vi "Report PDFCreator.vi"(0 "report in":refnum<class "NI_report.lvclass">, 2 "Conversion to PDF":enum16{"standard report", "file"}(ring), 7 "AutosaveDirectory":string="C:\\Users\\A Blaise\\Desktop\\Alouette\\Documents BD\\Rapports\\", 9 "AutosaveFilename":string="Allo", 11 "error in (no error)":errorcluster, 13 "Printer name":string="PDFCreator") -> (4 "report out":refnum<class "NI_report.lvclass">, 8 "More than 60 seconds":bool, 10 "File path":path, 15 "error out":errorcluster)   [LabVIEW 2010]
doc: "Jean-Marc Simard \nJanuary 6, 2010"
uses:
  <vilib>/Utility/NIReport.llb/NI_report.lvclass
panel:
  in  "File to convert":path
  in  "PDFCreator._clsPDFCreator":refnum<k7>
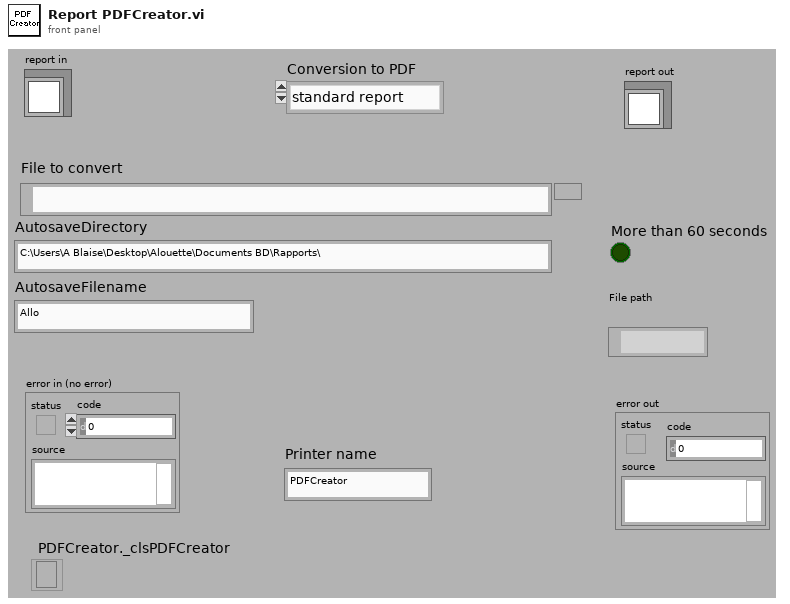
[diagram p1: front panel]
types:
  T1 = cluster{"UseAutosave":i32, "UseAutosaveDirectory":i32, "Autosave directory":string, "AutosaveFilename":string, "AutosaveFormat":i32}
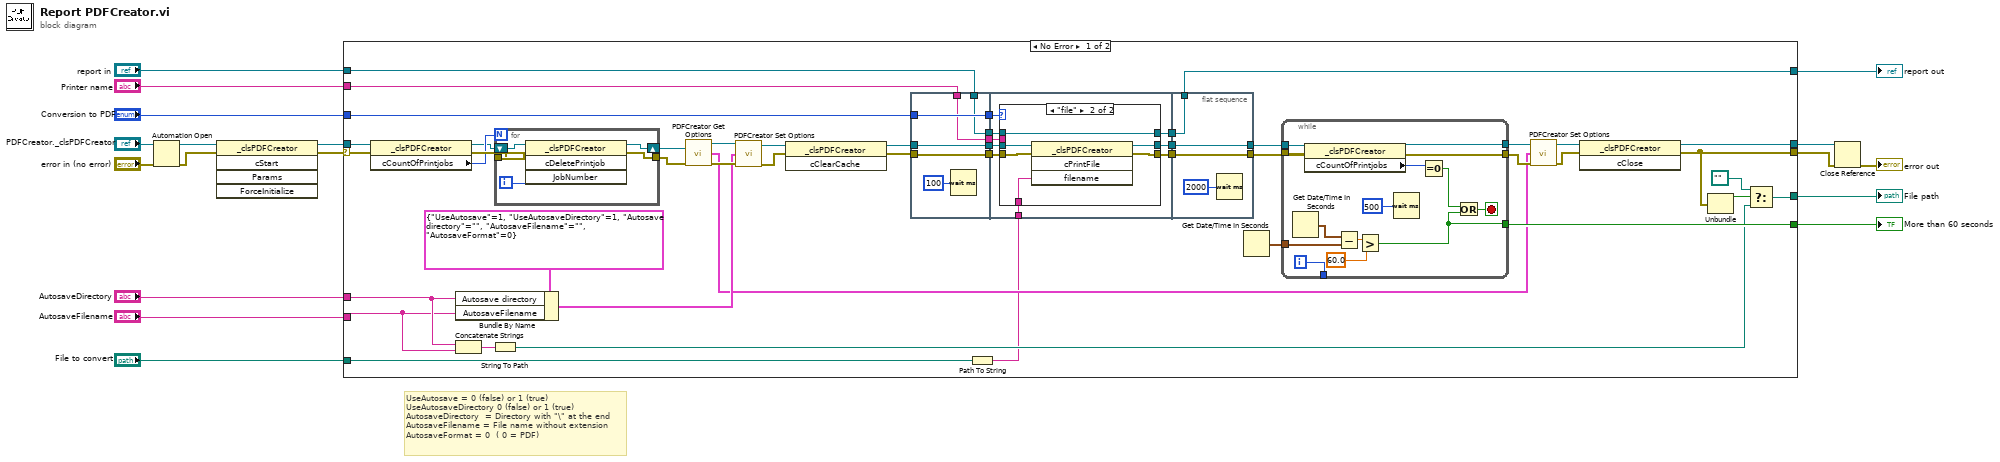
[diagram p0: block diagram]
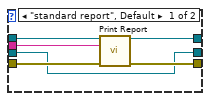
[diagram p2: hidden frame]
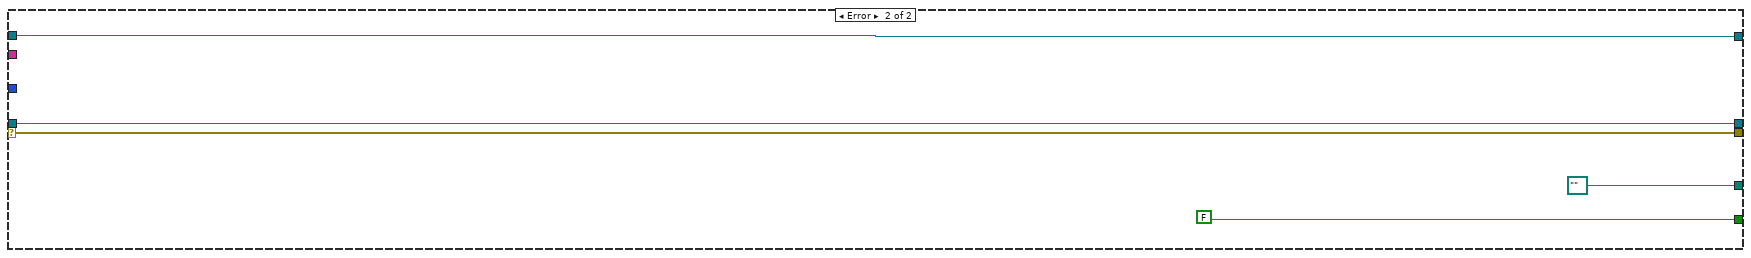
[diagram p3: hidden frame]
diagram:
  # "UseAutosave = 0 (false) or 1 (true)\nUseAutosaveDirectory 0 (false) or 1 (true)\nAutosaveDirectory  = Directory with \"\\\" at the end\nAutosaveFilename = File name without extension \nAutosaveFormat = 0  ( 0 = PDF)"
  n1 = Automation Open(error in (no error)="error in (no error)", Automation Refnum="PDFCreator._clsPDFCreator") -> (Automation Refnum=w7:refnum<k7>, error out=w17:errorcluster)  [unwired: 2 out]
  n2 = invoke class="_clsPDFCreator" method="cStart"(reference=w7, error in=w17) -> (reference out=w14:refnum<k7>, error out=w9:errorcluster)  [unwired: 3 in, 3 out]
  n3 = case shown="No Error" w9 {
    selector: w9 -> [w57 w119]
    tunnel: [w65 w120] -> w16
    tunnel: [w36 w119] -> w15
    tunnel: w14 -> [w63 w120]
    tunnel: "AutosaveDirectory" -> [w39 _]
    tunnel: "AutosaveFilename" -> [w38 _]
    tunnel: [w56 FALSE] -> w8
    tunnel: "report in" -> [w23 w117]
    tunnel: [w25 w117] -> w5
    tunnel: "Printer name" -> [w21 _]
    tunnel: [w33 path "" ("t")] -> w3
    tunnel: "Conversion to PDF" -> [w27 _]
    tunnel: "File to convert" -> [w19 _]
    frame No Error {
      n4 = property class="_clsPDFCreator"(reference=w63, error in=w57) -> (reference out=w58:refnum<k7>, error out=w60:errorcluster, "cCountOfPrintjobs"=w59:i32)
      n5 = Bundle By Name(cluster=T1 {"UseAutosave"=1, "UseAutosaveDirectory"=1, "Autosave directory"="", "AutosaveFilename"="", "AutosaveFormat"=0} ("Options"), "Autosave directory"=w39, "AutosaveFilename"=w38) -> (w45:T1)
      n6 = Concatenate Strings(w39, w38) -> (w37:string)
      n7 = String To Path(string=w37) -> (path=w29:path)
      n8 = for {
        N: w59 -> [_]
        tunnel: w60 -> [w99]
        tunnel: [w98] -> w55
        shift-right: [w101] -> w54
        shift-left: w58 -> [w100]
        i -> [w97]
        n9 = invoke class="_clsPDFCreator" method="cDeletePrintjob"(reference=w100, error in=w99, "JobNumber"=w97) -> (reference out=w101:refnum<k7>, error out=w98:errorcluster)  [unwired: 1 in, 2 out]
      }
      n10 = call "PDFCreator Get Options.vi"("PDFCreator._clsPDFCreator"=w54, "error in (no error)"=w55) -> ("PDFCreator._clsPDFCreator 2"=w52:refnum<k7>, "Options"=w40:T1, "error out"=w53:errorcluster)  [unwired: 11 out]
      n11 = call "PDFCreator Set Options.vi"("PDFCreator._clsPDFCreator"=w52, "Options"=w45, "error in (no error)"=w53) -> ("PDFCreator._clsPDFCreator 2"=w30:refnum<k7>, "error out"=w51:errorcluster)  [unwired: 11 out]
      n12 = invoke class="_clsPDFCreator" method="cClearCache"(reference=w30, error in=w51) -> (reference out=w61:refnum<k7>, error out=w62:errorcluster)  [unwired: 1 in, 1 out]
      n13 = flat-sequence {
        tunnel: w61 -> [w70]
        tunnel: w62 -> [w69]
        tunnel: [w70] -> w50
        tunnel: [w69] -> w49
        tunnel: w27 -> [w68]
        tunnel: [w68] -> w26
        tunnel: w23 -> [w67]
        tunnel: [w67] -> w22
        tunnel: w21 -> [w66]
        tunnel: [w66] -> w20
        tunnel: w50 -> [w77]
        tunnel: w49 -> [w80]
        tunnel: [w78] -> w32
        tunnel: [w79] -> w31
        tunnel: w28 -> [w76]
        tunnel: w26 -> [w75]
        tunnel: [w74] -> w24
        tunnel: w22 -> [w73]
        tunnel: w20 -> [w72]
        tunnel: [w95] -> w47
        tunnel: [w96] -> w48
        tunnel: w32 -> [w96]
        tunnel: w31 -> [w95]
        tunnel: [w93] -> w25
        tunnel: w24 -> [w93]
        frame #0 {
          n14 = Wait (ms)(milliseconds to wait=u32 100) -> ()  [unwired: 1 out]
        }
        frame #1 {
          n15 = case shown="\"file\"" w75 {
            tunnel: w80 -> [w86 w91]
            tunnel: [w85 w89] -> w79
            tunnel: [w84 w90] -> w78
            tunnel: w77 -> [w84 w92]
            tunnel: w76 -> [_ w88]
            tunnel: [w83 w87] -> w74
            tunnel: w73 -> [w82 w87]
            tunnel: w72 -> [w81 _]
            frame "standard report", Default {
              n16 = call-dynamic "Print Report.vi"("report in"=w82, "printer name (default)"=w81, "error in (no error)"=w86) -> ("report out"=w83:refnum<class "NI_report.lvclass">, "error out"=w85:errorcluster)  [unwired: 1 in, 10 out]
            }
            frame "file" {
              n17 = invoke class="_clsPDFCreator" method="cPrintFile"(reference=w92, error in=w91, "filename"=w88) -> (reference out=w90:refnum<k7>, error out=w89:errorcluster)  [unwired: 1 in, 2 out]
            }
          }
        }
        frame #2 {
          n18 = Wait (ms)(milliseconds to wait=u32 2000) -> ()  [unwired: 1 out]
        }
      }
      n19 = Path To String(path=w19) -> (string=w28:string)
      n20 = Get Date/Time In Seconds() -> (seconds since 1Jan1904=w64:timestamp)
      n21 = while {
        tunnel: w48 -> [w115]
        tunnel: w47 -> [w114]
        tunnel: [w113] -> w44
        tunnel: [w112] -> w43
        tunnel: w64 -> [w109]
        tunnel: [w103] -> w56
        tunnel: [w102] -> _
        i -> [w102]
        stop <- w104 stop-if-true
        n22 = Get Date/Time In Seconds() -> (seconds since 1Jan1904=w108:timestamp)
        n23 = property class="_clsPDFCreator"(reference=w115, error in=w114) -> (reference out=w113:refnum<k7>, error out=w112:errorcluster, "cCountOfPrintjobs"=w111:i32)
        n24 = Subtract(x=w108, y=w109) -> (x-y=w107:dbl)
        n25 = Greater?(x=w107, y=60.0) -> (0:w103:bool)
        n26 = Wait (ms)(milliseconds to wait=u32 500) -> ()  [unwired: 1 out]
        n27 = Equal To 0?(x=w111) -> (x = 0?=w105:bool)
        n28 = Or(x=w105, y=w103) -> (x .or. y?=w104:bool)
      }
      n29 = call "PDFCreator Set Options.vi"("PDFCreator._clsPDFCreator"=w44, "Options"=w40, "error in (no error)"=w43) -> ("PDFCreator._clsPDFCreator 2"=w42:refnum<k7>, "error out"=w41:errorcluster)  [unwired: 11 out]
      n30 = invoke class="_clsPDFCreator" method="cClose"(reference=w42, error in=w41) -> (reference out=w65:refnum<k7>, error out=w36:errorcluster)  [unwired: 1 in, 1 out]
      n31 = Unbundle(w36) -> ("status"=w35:bool)  [unwired: 2 out]
      n32 = Select(t=path "", s=w35, f=w29) -> (s? t:f=w33:path)
    }
    frame Error {
    }
  }
  "More than 60 seconds" <- w8
  "report out" <- w5
  "File path" <- w3
  n33 = Close Reference(reference=w16, error in (no error)=w15) -> (error out=→"error out":errorcluster)
